vi "SetParam.vi"(8 "error in (no error)":errorcluster caption="entrée d'erreur (pas d'erreur)", 10 "silhouette_score":T1={"metric"="euclidean", "sample_size"="None", "random_state"=-1} {"random_state" min=-1}, 11 "Silhouette_Score.lvclass":refnum<class "Silhouette_Score.lvclass">) -> (0 "error out":errorcluster caption="sortie d'erreur", 3 "Silhouette_Score.lvclass":refnum<class "Silhouette_Score.lvclass">)   [LabVIEW 2020, in "Silhouette_Score.lvclass"]
doc: "Set Parameters"
uses:
  Silhouette_Score.lvclass
  Silhouette_Score.lvclass/Silhouette_Score.ctl
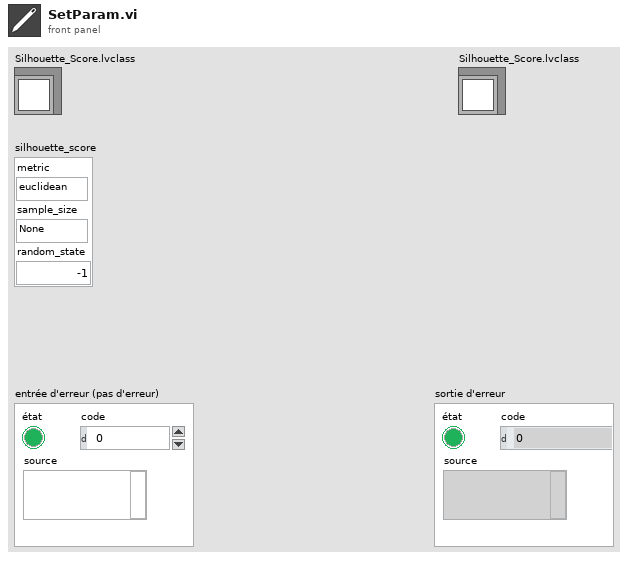
[diagram p1: front panel]
types:
  T1 = cluster{"metric":string, "sample_size":string, "random_state":i32}
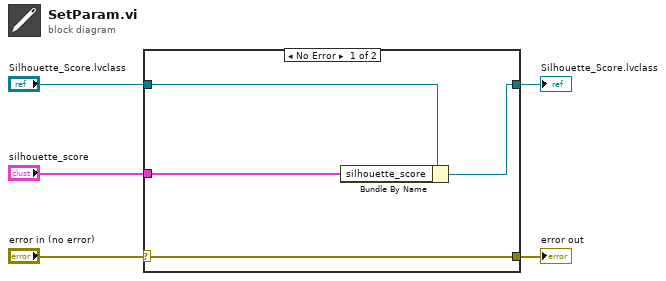
[diagram p0: block diagram]
diagram:
  n1 = case shown="No Error" "error in (no error)" {
    selector: "error in (no error)" -> [w9 w10]
    tunnel: [w9 w10] -> w4
    tunnel: [w7 w11] -> w2
    tunnel: "Silhouette_Score.lvclass" -> [w8 w11]
    tunnel: "silhouette_score" -> [w6 _]
    frame No Error {
      n2 = Bundle By Name(cluster=w8, "silhouette_score"=w6) -> (w7:refnum<class "Silhouette_Score.lvclass">)
    }
    frame Error {
    }
  }
  "error out" <- w4
  "Silhouette_Score.lvclass" <- w2
